vi "ExtractArmPositions.vi"(0 "Joint States":T2(array[cluster]), 1 "error in":errorcluster) -> (2 "left Positions":T1 {"w2" scale=-175.25..175.25; "w1" scale=-90.0..120.0; "w0" scale=-175.25..175.25; "e1" scale=-3.0..150.0; "e0" scale=-173.5..173.5; "s1" scale=-123.0..60.0; "s0" scale=-141.0..51.0}, 3 "right Positions":T1 {"w2" scale=-175.25..175.25; "w1" scale=-90.0..120.0; "w0" scale=-175.25..175.25; "e1" scale=-3.0..150.0; "e0" scale=-173.5..173.5; "s1" scale=-123.0..60.0; "s0" scale=-141.0..51.0}, 4 "error out":errorcluster)   [LabVIEW 2013]
doc: "Read all the current joint states (names, positions, velocity, and efforts)"
uses:
  ROS/Code/JointPositions.ctl
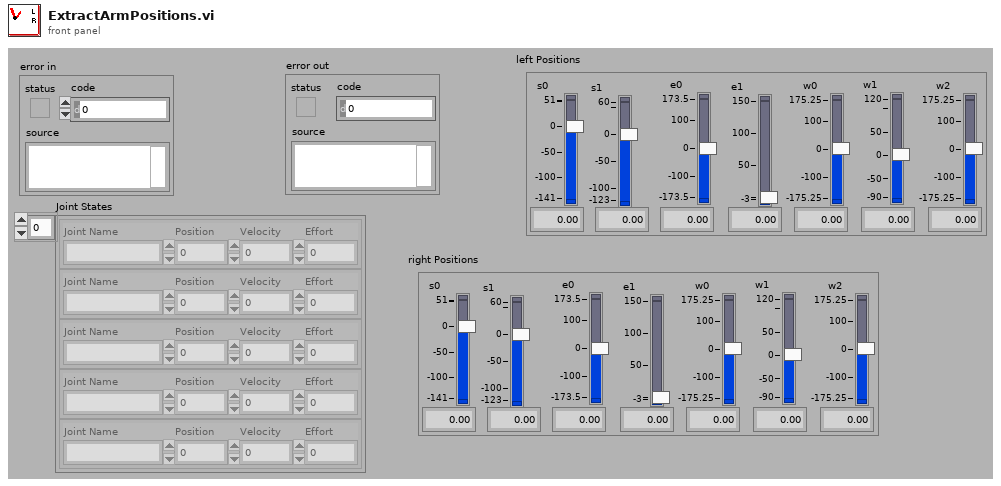
[diagram p1: front panel]
types:
  T1 = typedef "JointPositions.ctl" = cluster{"e0":dbl, "e1":dbl, "s0":dbl, "s1":dbl, "w0":dbl, "w1":dbl, "w2":dbl}
  T2 = cluster{"Joint Name":string, "Position":dbl, "Velocity":dbl, "Effort":dbl}[]
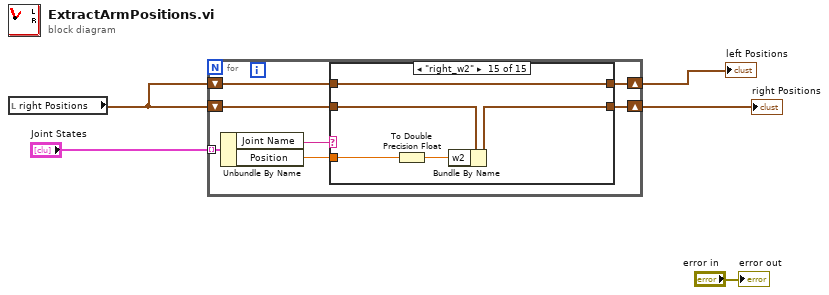
[diagram p0: block diagram]
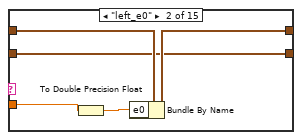
[diagram p3: hidden frame]
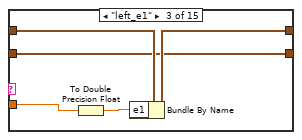
[diagram p4: hidden frame]
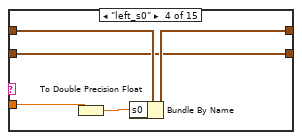
[diagram p5: hidden frame]
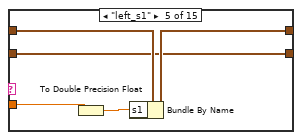
[diagram p6: hidden frame]
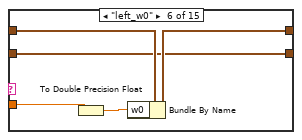
[diagram p7: hidden frame]
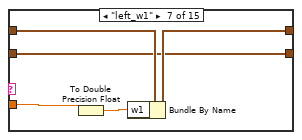
[diagram p8: hidden frame]
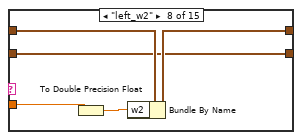
[diagram p9: hidden frame]
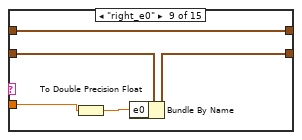
[diagram p10: hidden frame]
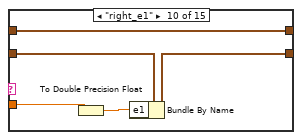
[diagram p11: hidden frame]
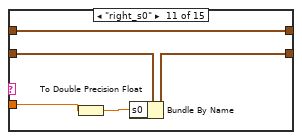
[diagram p12: hidden frame]
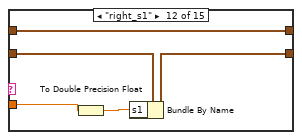
[diagram p13: hidden frame]
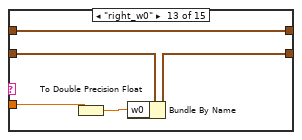
[diagram p14: hidden frame]
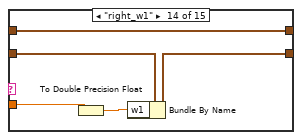
[diagram p15: hidden frame]
diagram:
  n1 = local read "right Positions"() -> (w1:T1)
  n2 = for {
    tunnel: "Joint States" -> [w12] mode=indexing
    shift-right: [w11] -> w2
    shift-left: w1 -> [w10]
    shift-right: [w6] -> w4
    shift-left: w1 -> [w7]
    n3 = Unbundle By Name(w12) -> ("Joint Name"=w9:string, "Position"=w8:dbl)
    n4 = case shown="\"right_w2\"" w9 {
      tunnel: [w14 w19 w24 w29 w34 w39 w44 w49 w50 w55 w60 w65 w70 w75 w80] -> w11
      tunnel: w10 -> [w14 w18 w23 w28 w33 w38 w43 w48 w50 w55 w60 w65 w70 w75 w80]
      tunnel: w8 -> [_ w16 w21 w26 w31 w36 w41 w46 w53 w58 w63 w68 w73 w78 w83]
      tunnel: w7 -> [w13 w15 w20 w25 w30 w35 w40 w45 w52 w57 w62 w67 w72 w77 w82]
      tunnel: [w13 w15 w20 w25 w30 w35 w40 w45 w51 w56 w61 w66 w71 w76 w81] -> w6
      frame Default {
      }
      frame "left_e0" {
        n5 = To Double Precision Float(number=w16) -> (double precision float=w17:dbl)
        n6 = Bundle By Name(cluster=w18, "e0"=w17) -> (w19:T1)
      }
      frame "left_e1" {
        n7 = To Double Precision Float(number=w21) -> (double precision float=w22:dbl)
        n8 = Bundle By Name(cluster=w23, "e1"=w22) -> (w24:T1)
      }
      frame "left_s0" {
        n9 = To Double Precision Float(number=w26) -> (double precision float=w27:dbl)
        n10 = Bundle By Name(cluster=w28, "s0"=w27) -> (w29:T1)
      }
      frame "left_s1" {
        n11 = To Double Precision Float(number=w31) -> (double precision float=w32:dbl)
        n12 = Bundle By Name(cluster=w33, "s1"=w32) -> (w34:T1)
      }
      frame "left_w0" {
        n13 = To Double Precision Float(number=w36) -> (double precision float=w37:dbl)
        n14 = Bundle By Name(cluster=w38, "w0"=w37) -> (w39:T1)
      }
      frame "left_w1" {
        n15 = To Double Precision Float(number=w41) -> (double precision float=w42:dbl)
        n16 = Bundle By Name(cluster=w43, "w1"=w42) -> (w44:T1)
      }
      frame "left_w2" {
        n17 = To Double Precision Float(number=w46) -> (double precision float=w47:dbl)
        n18 = Bundle By Name(cluster=w48, "w2"=w47) -> (w49:T1)
      }
      frame "right_e0" {
        n19 = To Double Precision Float(number=w53) -> (double precision float=w54:dbl)
        n20 = Bundle By Name(cluster=w52, "e0"=w54) -> (w51:T1)
      }
      frame "right_e1" {
        n21 = To Double Precision Float(number=w58) -> (double precision float=w59:dbl)
        n22 = Bundle By Name(cluster=w57, "e1"=w59) -> (w56:T1)
      }
      frame "right_s0" {
        n23 = To Double Precision Float(number=w63) -> (double precision float=w64:dbl)
        n24 = Bundle By Name(cluster=w62, "s0"=w64) -> (w61:T1)
      }
      frame "right_s1" {
        n25 = To Double Precision Float(number=w68) -> (double precision float=w69:dbl)
        n26 = Bundle By Name(cluster=w67, "s1"=w69) -> (w66:T1)
      }
      frame "right_w0" {
        n27 = To Double Precision Float(number=w73) -> (double precision float=w74:dbl)
        n28 = Bundle By Name(cluster=w72, "w0"=w74) -> (w71:T1)
      }
      frame "right_w1" {
        n29 = To Double Precision Float(number=w78) -> (double precision float=w79:dbl)
        n30 = Bundle By Name(cluster=w77, "w1"=w79) -> (w76:T1)
      }
      frame "right_w2" {
        n31 = To Double Precision Float(number=w83) -> (double precision float=w84:dbl)
        n32 = Bundle By Name(cluster=w82, "w2"=w84) -> (w81:T1)
      }
    }
  }
  "right Positions" <- w4
  "left Positions" <- w2
  "error out" <- "error in"
